vi "pxi cpu check.vi"() -> ()   [LabVIEW 2014]
uses:
  <vilib>/Platform/TimedLoop/XDataNode/timing_clust.ctl
  <vilib>/Platform/TimedLoop/XDataNode/nitl_modes.ctl
  <vilib>/Platform/TimedLoop/XDataNode/wakeup.ctl
  <vilib>/Utility/file.llb/Write To Spreadsheet File (DBL).vi
  <vilib>/Platform/TimedLoop/XDataNode/XDataNode.xnode
  <vilib>/Platform/TimedLoop/XDataNode/XDNodeRunTimeDep.lvlib
panel:
  in  "Boolean":bool
  out "Waveform Chart":T1(graph)
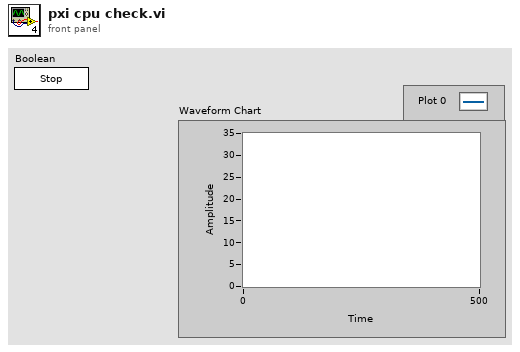
[diagram p1: front panel]
types:
  T1 = cluster{"[0]":dbl, "[1]":dbl, "[2]":dbl, "[3]":dbl}
  T2 = typedef "XDNodeRunTimeDep.lvlib/timing_clust.ctl" = cluster{"Expected End [f-1]":u64, "Actual End [f-1]":u64, "Finished Late? [f-1]":bool, "Expected End [i-1]":u64, "Actual End [i-1]":u64, "Finished Late? [i-1]":bool, "Expected Start [i]":u64, "Actual Start [i]":u64, "Expected Start [f]":u64, "Actual Start [f]":u64, "Source Name":string, "Structure Name":string, "Period":i64, "Deadline":i64, "Offset":i64, "Start":i64, "Priority":i32, "Timeout":i32, "Mode":T3, "Wakeup Reason":T4, "Error":errorcluster, "Source Type":string, "Secondary Source Type":string, "Global End Time":u64, "Global Start Time":u64, "Frame Duration":u64, "Iteration Duration":u64, "Assigned CPU":i32, "I/O Scan Engine Mode":u32}
  T3 = typedef "XDNodeRunTimeDep.lvlib/nitl_modes.ctl" = enum32{"No Change", "Process missed periods, maintain original phase", "Discard missed periods, maintain original phase", "Process missed periods, ignore original phase", "Discard missed periods, ignore original phase"}
  T4 = typedef "XDNodeRunTimeDep.lvlib/wakeup.ctl" = enum32{"Normal", "Aborted", "Asynchronous wakeup", "Timing source error", "Timed loop error", "Timeout"}
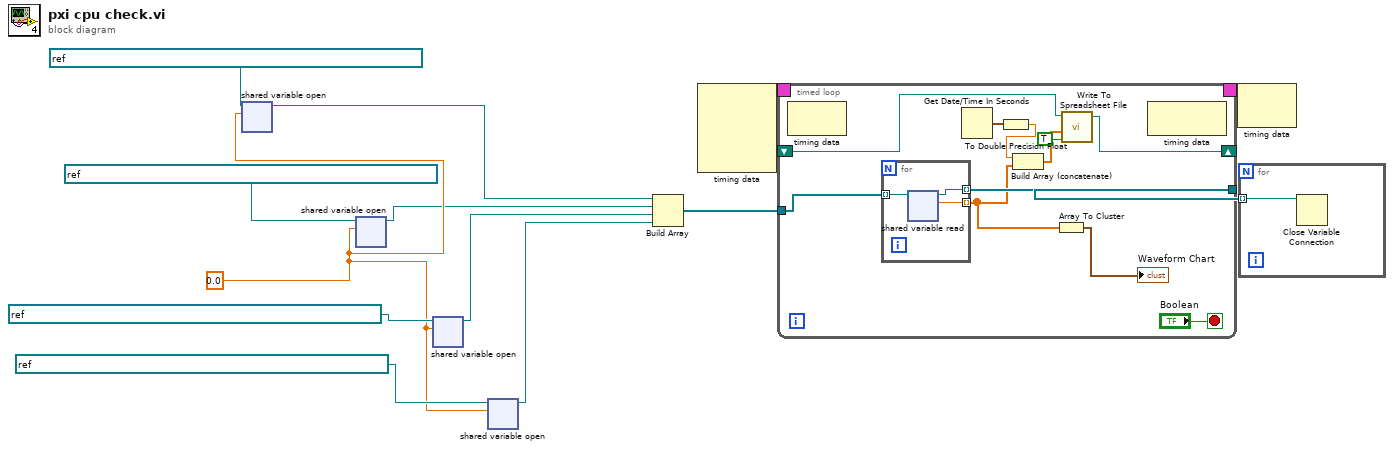
[diagram p0: block diagram]
diagram:
  w9 = 0.0
  n1 = shared-variable-open(refnum<k21> "ni.var.psp://10.172.240.106/NI_SystemState/CPULoad/CPU0/Total" ("shared variable refnum in"), w9) -> (w8:refnum<k21>)  [unwired: 2 in, 1 out]
  n2 = shared-variable-open(refnum<k21> "ni.var.psp://10.172.240.106/NI_SystemState/CPULoad/CPU1/Total" ("shared variable refnum in"), w9) -> (w7:refnum<k21>)  [unwired: 2 in, 1 out]
  n3 = shared-variable-open(refnum<k21> "ni.var.psp://10.172.240.106/NI_SystemState/CPULoad/CPU2/Total" ("shared variable refnum in"), w9) -> (w6:refnum<k21>)  [unwired: 2 in, 1 out]
  n4 = shared-variable-open(refnum<k21> "ni.var.psp://10.172.240.106/NI_SystemState/CPULoad/CPU3/Total" ("shared variable refnum in"), w9) -> (w5:refnum<k21>)  [unwired: 2 in, 1 out]
  n5 = Build Array(w8, w7, w6, w5) -> (w4:refnum<k21>[])
  n6 = node-c288() -> (w2:T2)  [unwired: 4 in]
  n7 = timed-loop {
    tunnel: w4 -> [w24]
    tunnel: [w23] -> w3
    timing: w2 -> [_]
    timing-out: [_] -> w1
    shift-right: [w16] -> _
    shift-left: _ -> [w15]
    stop <- "Boolean" stop-if-true
    n8 = node-c288() -> ()  [unwired: 1 in, 1 out]
    n9 = for {
      tunnel: w24 -> [w29] mode=indexing
      tunnel: [w28] -> w20 mode=indexing
      tunnel: [w27] -> w23 mode=indexing
      n10 = shared-variable-read(w29) -> (w27:refnum<k21>, w28:dbl)  [unwired: 1 in, 2 out]
    }
    n11 = Get Date/Time In Seconds() -> (seconds since 1Jan1904=w19:timestamp)
    n12 = To Double Precision Float(number=w19) -> (double precision float=w18:dbl)
    n13 = Build Array (concatenate)(w18, w20) -> (w17:dbl[])
    n14 = Array To Cluster(array=w20) -> (cluster=→"Waveform Chart":T1)
    n15 = call-poly <vilib>:"Write To Spreadsheet File.vi"("append to file? (new file:F)"=TRUE, "1D data"=w17, "file path (dialog if empty)"=w15) -> ("new file path (Not A Path if cancelled)"=w16:path)  [unwired: 5 in]
    n16 = node-c288() -> ()  [unwired: 1 in, 1 out]
  }
  n17 = node-c288(w1) -> ()  [unwired: 1 out]
  n18 = for {
    tunnel: w3 -> [w30] mode=indexing
    n19 = Close Variable Connection(11:w30) -> ()  [unwired: 1 in, 1 out]
  }
